vi "Configuration.vi"(6 "Return Data":refnum<user-event>, 8 "error in (no error)":errorcluster, 9 "Exit Running Config":refnum<user-event>, 10 "Panel in":refnum<class "Panel.lvclass">, 11 "Boolean Data Type in":refnum<class "Boolean Data Type.lvclass">) -> (0 "error out":errorcluster, 3 "Boolean Data Type out":refnum<class "Boolean Data Type.lvclass">)   [LabVIEW 2018, in "Boolean Data Type.lvclass"]
uses:
  Boolean Data Type.lvclass
  D:/Code/QControls Extended/DataGrid/DataGrid Configuration/Data Type Classes/Generic/Generic Data Type.lvclass
  <vilib>/MGI/Panel Manager/Panel/Panel/Panel.lvclass
  Generic/Generic Data Type.lvclass
  Value Pairs.ctl
  Boolean Data Type.lvclass/Boolean Data Type.ctl
  Generic/Generic Data Type.lvclass/Generic Data Type.ctl
  Generic/Write Column Header.vi
  Generic/Read Column Header.vi
panel:
  in  "Column Header":string
  in  "False String":string
  in  "True String":string
  in  "Default Value":bool
  in  "Value Pairs":T1
  # "Boolean Column"
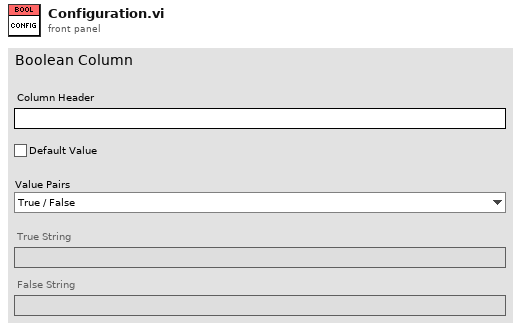
[diagram p1: front panel]
types:
  T1 = typedef "Boolean Data Type.lvclass/Value Pairs.ctl" = enum16{"True / False", "Yes / No", "X / [Blank]", "On / Off", "Custom"}
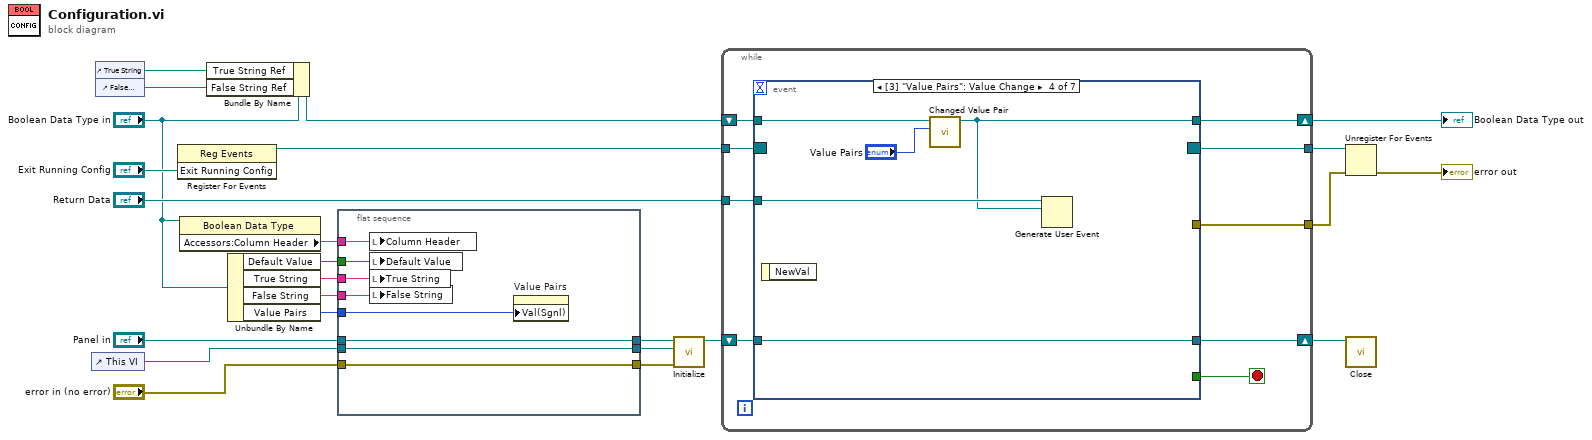
[diagram p0: block diagram]
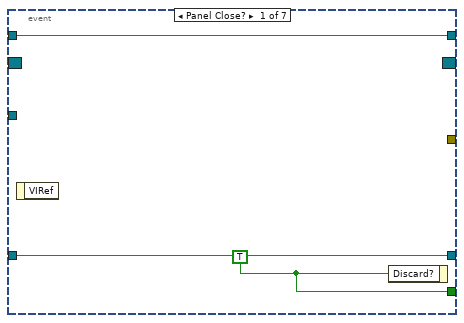
[diagram p2: hidden frame]
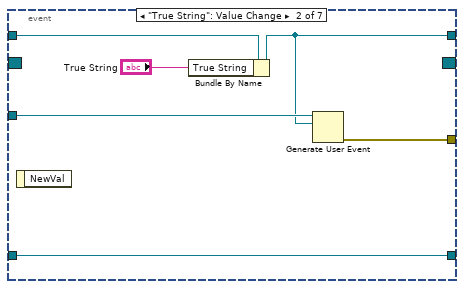
[diagram p3: hidden frame]
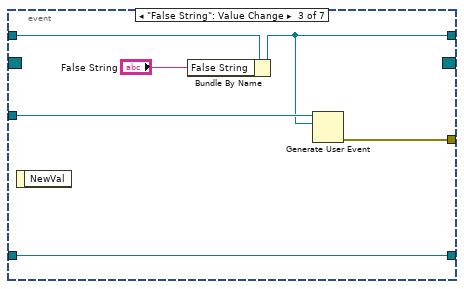
[diagram p4: hidden frame]
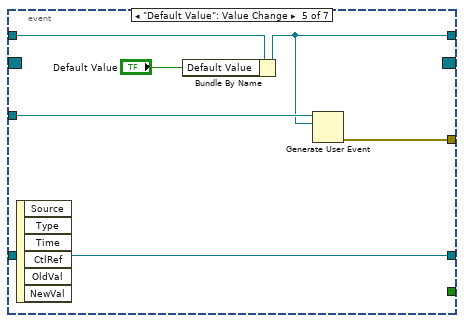
[diagram p5: hidden frame]
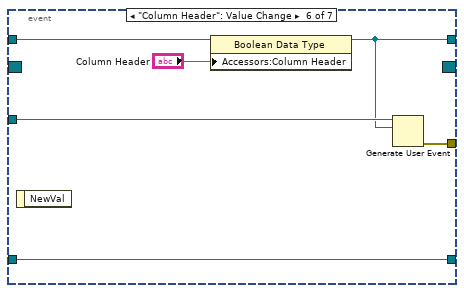
[diagram p6: hidden frame]
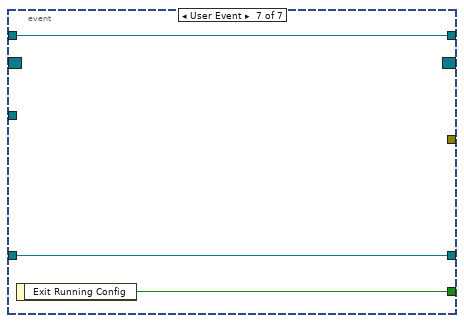
[diagram p7: hidden frame]
diagram:
  n1 = control-ref of="This VI"() -> (w20:refnum<vi>)
  n2 = control-ref of="True String"() -> (w4:refnum<vi>)
  n3 = control-ref of="False String"() -> (w5:refnum<vi>)
  n4 = register-events("Exit Running Config") -> (reference out=w14:refnum<event-registration>)  [unwired: 2 in, 1 out]
  n5 = property class="Boolean Data Type"(reference="Boolean Data Type in") -> ("Accessors:Column Header"=w24:string)  [unwired: 1 in, 2 out]
  n6 = Bundle By Name(cluster="Boolean Data Type in", "True String Ref"=w4, "False String Ref"=w5) -> (w2:refnum<class "Boolean Data Type.lvclass">)
  n7 = Unbundle By Name("Boolean Data Type in") -> ("Default Value"=w23:bool, "True String"=w17:string, "False String"=w9:string, "Value Pairs"=w1:T1)
  n8 = flat-sequence {
    tunnel: w17 -> [w32]
    tunnel: "Panel in" -> [w31]
    tunnel: [w31] -> w18
    tunnel: [w30] -> w19
    tunnel: w20 -> [w30]
    tunnel: "error in (no error)" -> [w29]
    tunnel: [w29] -> w22
    tunnel: w23 -> [w28]
    tunnel: w24 -> [w27]
    tunnel: w9 -> [w26]
    tunnel: w1 -> [w25]
    frame #0 {
      n9 = local write "Column Header"(w27) -> ()
      n10 = local write "Default Value"(w28) -> ()
      n11 = local write "True String"(w32) -> ()
      n12 = local write "False String"(w26) -> ()
      n13 = property on="Value Pairs" class="Enum (strict)"("Val(Sgnl)"=w25) -> ()  [unwired: 2 in, 2 out]
    }
  }
  n14 = call <vilib>:"Initialize.vi"("error in (no error)"=w22, "VI Refnum"=w19, "Panel In"=w18) -> ("Panel Out"=w16:refnum<class "Panel.lvclass">)  [unwired: 6 in, 2 out]
  n15 = while {
    shift-right: [w35] -> w12
    shift-left: w2 -> [w41]
    shift-right: [w37] -> w15
    shift-left: w16 -> [w38]
    tunnel: w14 -> [w39]
    tunnel: [w36] -> w13
    tunnel: "Return Data" -> [w34]
    tunnel: [w33] -> w21
    stop <- w40 stop-if-true
    n16 = event shown="[3] \"Value Pairs\": Value Change" {
      selector: w39 -> [_ _ _ _ _ _ _]
      dyn-events: [_ _ _ _ _ _ _] -> w36
      timeout: _ -> [_ _ _ _ _ _ _]
      tunnel: w41 -> [w44 w49 w55 w60 w66 w70 w76]
      tunnel: [w44 w47 w53 w57 w64 w69 w76] -> w35
      tunnel: [w43 _ _ _ _ _ w75] -> w40
      tunnel: w38 -> [w42 w50 w56 w61 w67 w73 w74]
      tunnel: [w42 w50 w56 w61 w67 w73 w74] -> w37
      tunnel: w34 -> [_ w48 w54 w58 w65 w72 _]
      tunnel: [_ w46 w52 _ w63 w71 _] -> w33
      event Panel Close? {
        w43 = TRUE
        n17 = event-data() -> ()  [unwired: 1 in, 1 out]
        n18 = event-data("Discard?"=w43) -> ()  [unwired: 1 in, 1 out]
      }
      event "True String": Value Change {
        n19 = event-data() -> ()  [unwired: 1 in, 1 out]
        n20 = Bundle By Name(cluster=w49, "True String"="True String") -> (w47:refnum<class "Boolean Data Type.lvclass">)
        n21 = Generate User Event(user event=w48, event data cluster=w47) -> (error out=w46:errorcluster)  [unwired: 2 in, 1 out]
      }
      event "False String": Value Change {
        n22 = event-data() -> ()  [unwired: 1 in, 1 out]
        n23 = Bundle By Name(cluster=w55, "False String"="False String") -> (w53:refnum<class "Boolean Data Type.lvclass">)
        n24 = Generate User Event(user event=w54, event data cluster=w53) -> (error out=w52:errorcluster)  [unwired: 2 in, 1 out]
      }
      event Value Change {
        n25 = event-data() -> ()  [unwired: 1 in, 1 out]
        n26 = call "Changed Value Pair.vi"("Value Pairs"="Value Pairs", "Boolean Data Type in"=w60) -> ("Boolean Data Type out"=w57:refnum<class "Boolean Data Type.lvclass">)  [unwired: 8 in, 1 out]
        n27 = Generate User Event(user event=w58, event data cluster=w57) -> ()  [unwired: 2 in, 2 out]
      }
      event "Default Value": Value Change {
        n28 = event-data() -> ()  [unwired: 1 in, 6 out]
        n29 = Bundle By Name(cluster=w66, "Default Value"="Default Value") -> (w64:refnum<class "Boolean Data Type.lvclass">)
        n30 = Generate User Event(user event=w65, event data cluster=w64) -> (error out=w63:errorcluster)  [unwired: 2 in, 1 out]
      }
      event "Column Header": Value Change {
        n31 = event-data() -> ()  [unwired: 1 in, 1 out]
        n32 = property class="Boolean Data Type"(reference=w70, "Accessors:Column Header"="Column Header") -> (reference out=w69:refnum<class "Boolean Data Type.lvclass">)  [unwired: 1 in, 1 out]
        n33 = Generate User Event(user event=w72, event data cluster=w69) -> (error out=w71:errorcluster)  [unwired: 2 in, 1 out]
      }
      event User Event {
        n34 = event-data() -> ("Exit Running Config"=w75:bool)  [unwired: 1 in]
      }
    }
  }
  "Boolean Data Type out" <- w12
  n35 = Unregister For Events(event registration refnum=w13, error in=w21) -> (error out=→"error out":errorcluster)
  n36 = call-dynamic "Close.vi"("Panel In"=w15) -> ()  [unwired: 10 in, 1 out]
